vi "Checkers PvC.vi"() -> (9 "String 2":string="Player 2", 10 "String":string="Player 1")   [LabVIEW 2016]
panel:
  out "String 5":string
  out "Your Turn!":bool
  out "Your Turn!":bool
  out "String 4":string="Player 1"
  out "String 3":string="Player 1"
  in  "OK Button 3":bool
  in  "OK Button 2":bool
  in  "OK Button":bool
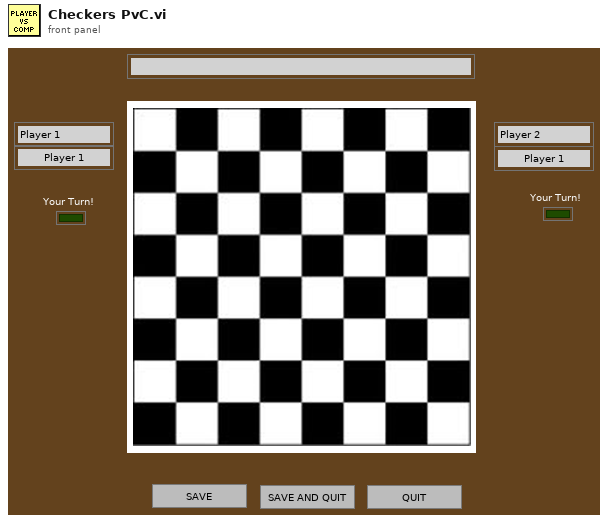
[diagram p1: front panel]
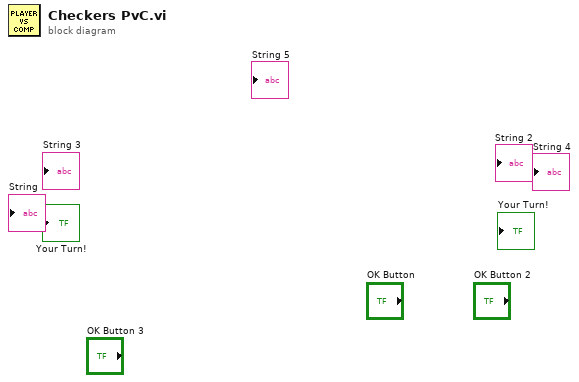
[diagram p0: block diagram]
diagram:
